vi "Kinesis - KPZ101 - Connect.vi"() -> ()   [LabVIEW 2012]
uses:
  U:/Kinesis LabVIEW Website Examples/Thorlabs.MotionControl.Controls.dll
  Thorlabs.MotionControl.Controls.dll
panel:
  in  "?":bool
  in  "SerialNumber":string
  in  "KCubePiezoControl":refnum<k24>(container)
  # "Notes:"
  # "- Ensure that the appropriate .DLLs are copied into your Project Folder. Check that the correct bit type are used depending on your version of LabVIEW\ni.e. 32-bit or 64-bit.\n\n\n\n\n\n\n\n\n\n\n\n\n\n\n- Open the example VI through the LabVIEW Project Explorer to correctly load the User Interface from Thorlabs.MotionControl.Controls.dll."
  # "Thorlabs Hardware: KPZ101 - K-Cube Piezo Controller\nhttps://www.thorlabs.com/newgrouppage9.cfm?objectgroup_id=2421&pn=KPZ101\n\nDescription: This VI shows you how to initialize communication with and then disconnect the KPZ101 Piezo controller.\n\nInstructions: \n1) Connect your KPZ101 device to your PC & power the device.\nFor full device setup, the device product manual can be found on our website here. - https://www.thorlabs.com/thorproduct.cfm?partnumber=KPZ101\n2) Enter the device serial number below.\n3) Click 'Run' in the LabVIEW Toolbar.\n4) To End the progam, click the 'STOP' button."
  # "Example Image of .NET Controller - VI opened via Project Explorer/ not opened via Project Explorer"
  # "VI Not Opened via Project Explorer"
  # "VI Opened via Project Explorer"
  # "- To explore the range of methods available, please visit the .NET API, included with your Kinesis software.\n\n- For tips on building your own VIs with Thorlabs Motion Control Hardware, please see our LabVIEW Guide here.\nhttps://www.thorlabs.com/newgrouppage9.cfm?objectgroup_id=10285"
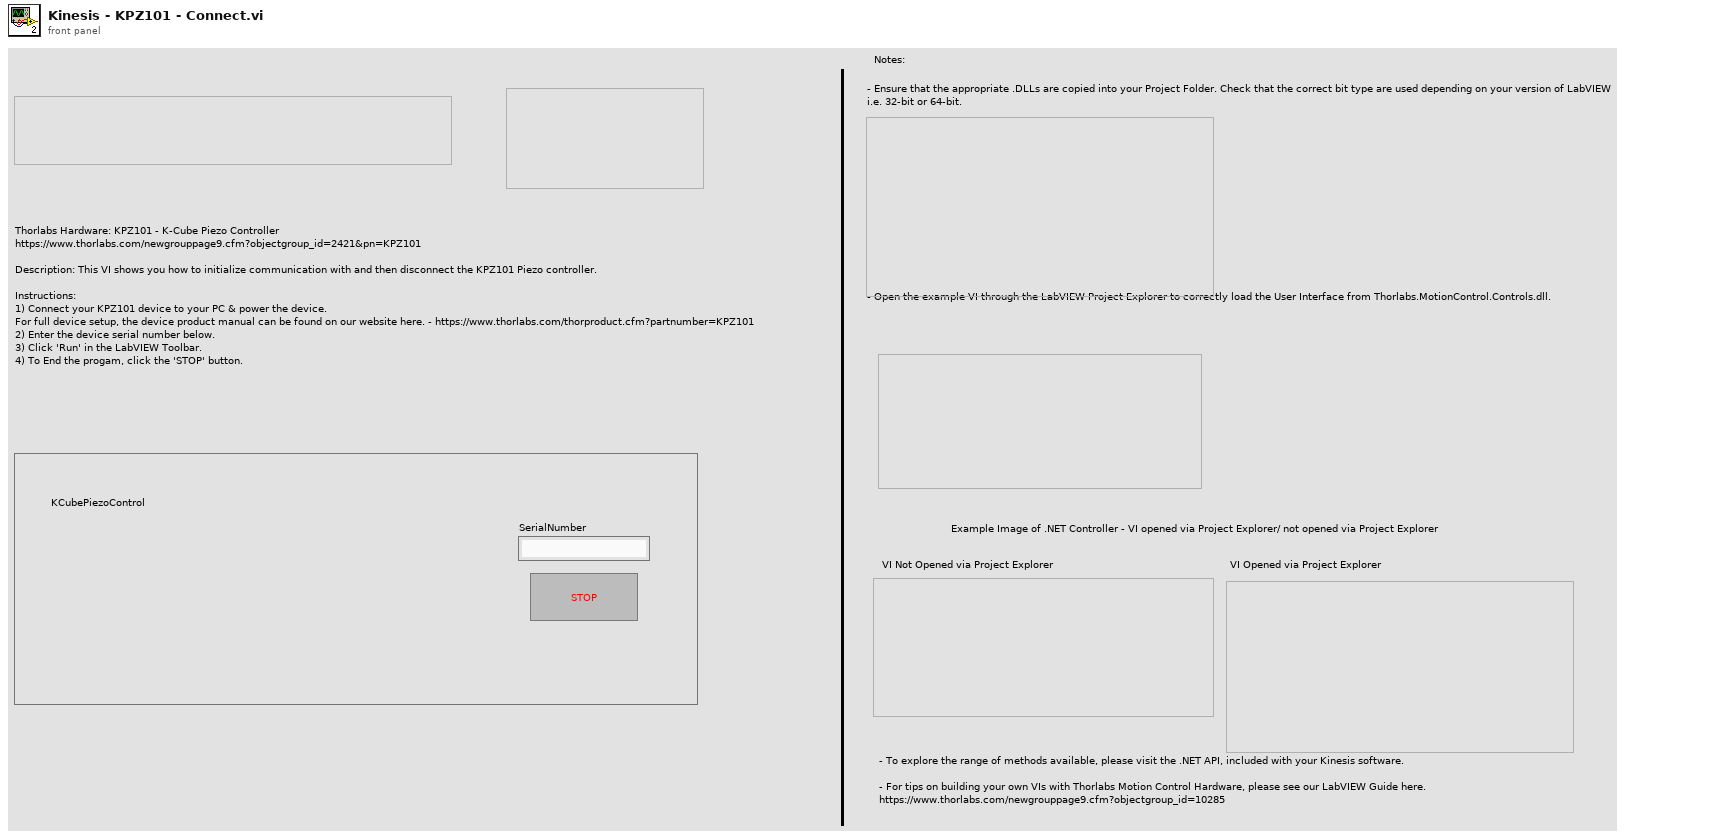
[diagram p1: front panel]
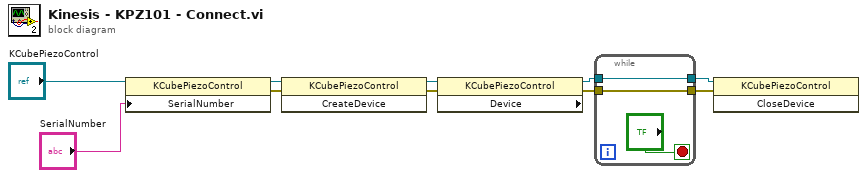
[diagram p0: block diagram]
diagram:
  n1 = property class="KCubePiezoControl"(reference="KCubePiezoControl", "SerialNumber"="SerialNumber") -> (reference out=w8:refnum<k24>, error out=w7:errorcluster)  [unwired: 1 in]
  n2 = invoke class="KCubePiezoControl" method="CreateDevice"(reference=w8, error in=w7) -> (reference out=w6:refnum<k24>, error out=w5:errorcluster)  [unwired: 1 in, 1 out]
  n3 = property class="KCubePiezoControl" props=["Device"](reference=w6, error in=w5) -> (reference out=w3:refnum<k24>, error out=w1:errorcluster)  [unwired: 1 out]
  n4 = while {
    tunnel: [w12] -> w4
    tunnel: w3 -> [w12]
    tunnel: [w11] -> w2
    tunnel: w1 -> [w11]
    stop <- "?" stop-if-true
  }
  n5 = invoke class="KCubePiezoControl" method="CloseDevice"(reference=w4, error in=w2) -> ()  [unwired: 1 in, 3 out]
